vi "Fit VI window to Pane Center.vi"(4 "Error In":errorcluster, 6 "Pane Ref":refnum<vi>, 7 "VI Ref (calling VI)":refnum<vi>) -> (0 "Error Out":errorcluster, 3 "dup VI Ref":refnum<vi>)   [LabVIEW 2017]
doc: "This VI is designed to center a callee VI's window in a caller VI's window.\n\nAuthored by Brandon Steele\nsupport@mooregoodideas.com\nwww.mooregoodideas.com\n\nCopyright (c) 2010, Moore Good Ideas, Inc.\n\nAll rights reserved.\n\nRedistribution and use in source and binary forms, with or without modification, are permitted provided that the following conditions are met:\n\n * Redistributions of source code must retain the above copyright notice, this list of conditions and the following disclaimer.\n * Redistributions in binary form must reproduce the above copyright notice, this list of conditions and the following disclaimer in the documentation and/or other materials provided with the distribution.\n * Neither the name of Moore Good Ideas, Inc. nor the names of its contributors may be used to endorse or promote products derived from this software without specific prior written permission.\n\nTHIS SOFTWARE IS PROVIDED BY THE COPYRIGHT HOLDERS AND CONTRIBUTORS \"AS IS\" AND ANY EXPRESS OR IMPLIED WARRANTIES, INCLUDING, BUT NOT LIMITED TO, THE IMPLIED WARRANTIES OF MERCHANTABILITY AND FITNESS FOR A PARTICULAR PURPOSE ARE DISCLAIMED. IN NO EVENT SHALL THE COPYRIGHT OWNER OR CONTRIBUTORS BE LIABLE FOR ANY DIRECT, INDIRECT, INCIDENTAL, SPECIAL, EXEMPLARY, OR CONSEQUENTIAL DAMAGES (INCLUDING, BUT NOT LIMITED TO, PROCUREMENT OF SUBSTITUTE GOODS OR SERVICES; LOSS OF USE, DATA, OR PROFITS; OR BUSINESS INTERRUPTION) HOWEVER CAUSED AND ON ANY THEORY OF LIABILITY, WHETHER IN CONTRACT, STRICT LIABILITY, OR TORT (INCLUDING NEGLIGENCE OR OTHERWISE) ARISING IN ANY WAY OUT OF THE USE OF THIS SOFTWARE, EVEN IF ADVISED OF THE POSSIBILITY OF SUCH DAMAGE."
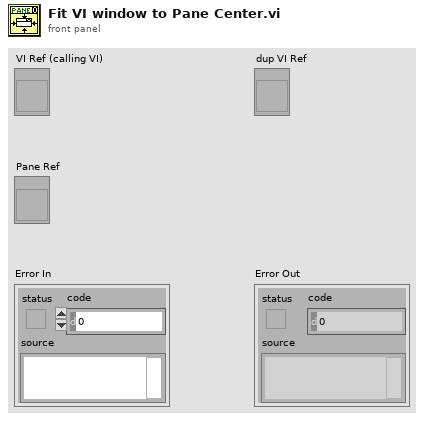
[diagram p1: front panel]
types:
  T1 = typedef "LVRectTypeDef.ctl" = cluster{"Left":i16, "Top":i16, "Right":i16, "Bottom":i16}
  T2 = cluster{"left":i16, "top":i16, "right":i16, "bottom":i16}
  T3 = typedef "LVAllMonitorsDisplayTypeDef.ctl" = cluster{"Bounds":cluster{"Left":i16, "Top":i16, "Right":i16, "Bottom":i16}, "Depth":i16}[]
  T4 = cluster{"Left":i16, "Top":i16, "Right":i16, "Bottom":i16}
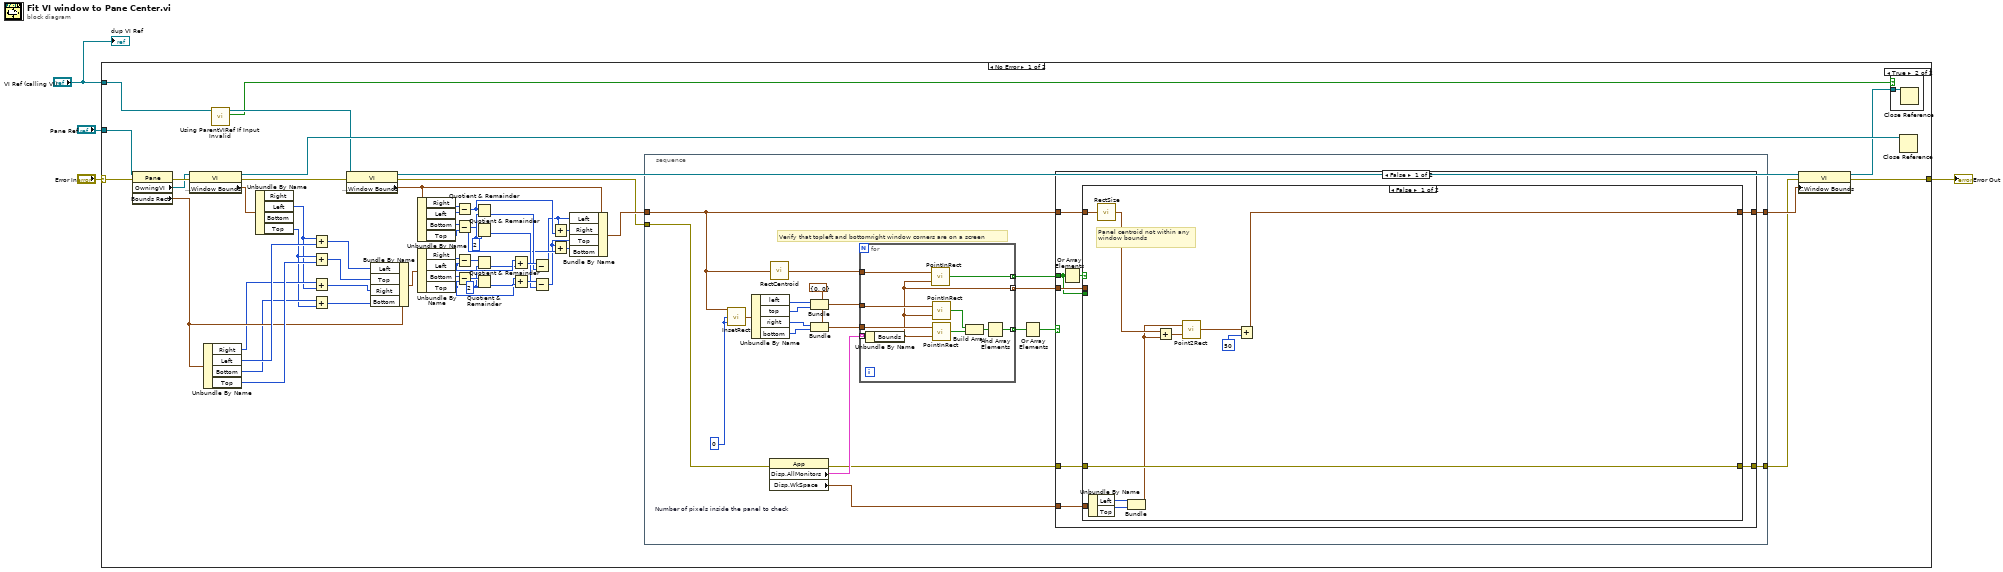
[diagram p0: block diagram]
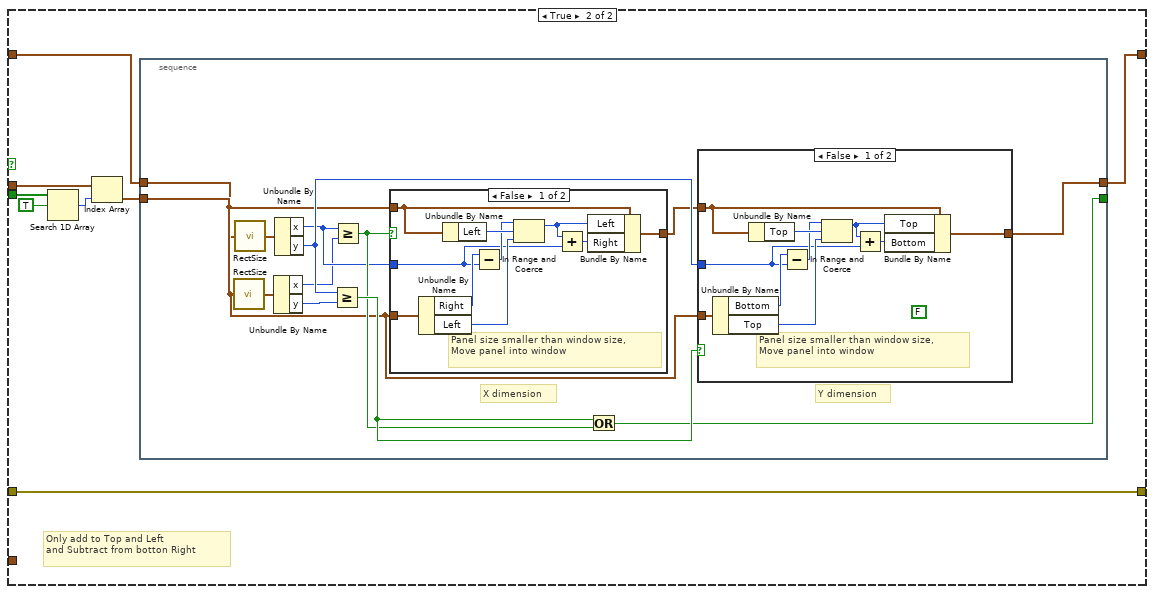
[diagram p2: hidden frame]
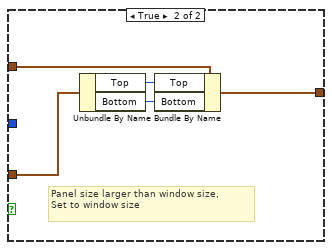
[diagram p3: hidden frame]
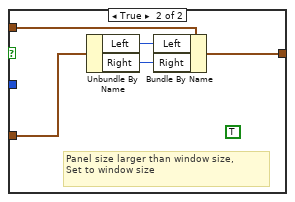
[diagram p4: hidden frame]
diagram:
  n1 = case shown="No Error" "Error In" {
    selector: "Error In" -> [w21 w163]
    tunnel: [w58 w163] -> w4
    tunnel: "Pane Ref" -> [w15 _]
    tunnel: "VI Ref (calling VI)" -> [w35 _]
    frame No Error {
      w52 = i16 2 ("y")
      w36 = i16 2 ("y")
      n2 = property class="Pane"(reference=w15, error in=w21) -> (error out=w20:errorcluster, "OwningVI"=w19:refnum<vi>, "Bounds Rect"=w12:T1)  [unwired: 1 out]
      n3 = property class="VI"(reference=w19, error in=w20) -> (reference out=w34:refnum<vi>, error out=w53:errorcluster, "Front Panel Window:Window Bounds"=w18:T1)
      n4 = Unbundle By Name(w12) -> ("Right"=w9:i16, "Left"=w14:i16, "Bottom"=w8:i16, "Top"=w13:i16)
      n5 = call "Using ParentVIRef If Input Invalid.vi"("VI Ref (calling VI)"=w35) -> ("Using Parent Ref(Need to Destroy)"=w24:bool, "VI Ref"=w32:refnum<vi>)  [unwired: 5 in]
      n6 = Unbundle By Name(w18) -> ("Left"=w6:i16, "Top"=w7:i16)  [unwired: 2 out]
      n7 = Add(x=w6, y=w14) -> (x+y=w17:i16)
      n8 = Add(x=w7, y=w13) -> (x+y=w16:i16)
      n9 = Add(x=w9, y=w6) -> (x+y=w11:i16)
      n10 = Add(x=w8, y=w7) -> (x+y=w10:i16)
      n11 = property class="VI"(reference=w32, error in=w53) -> (reference out=w39:refnum<vi>, error out=w23:errorcluster, "Front Panel Window:Window Bounds"=w27:T1)
      n12 = Bundle By Name(cluster=w12, "Left"=w17, "Top"=w16, "Right"=w11, "Bottom"=w10) -> (w5:T1)
      n13 = Unbundle By Name(w27) -> ("Right"=w48:i16, "Left"=w49:i16, "Bottom"=w50:i16, "Top"=w51:i16)
      n14 = Unbundle By Name(w5) -> ("Right"=w57:i16, "Left"=w47:i16, "Bottom"=w56:i16, "Top"=w44:i16)
      n15 = Subtract(x=w48, y=w49) -> (x-y=w38:i16)
      n16 = Subtract(x=w50, y=w51) -> (x-y=w37:i16)
      n17 = Subtract(x=w57, y=w47) -> (x-y=w55:i16)
      n18 = Subtract(x=w56, y=w44) -> (x-y=w54:i16)
      n19 = Quotient & Remainder(x=w38, y=w52) -> (floor(x/y)=w42:i16)  [unwired: 1 out]
      n20 = Quotient & Remainder(x=w37, y=w52) -> (floor(x/y)=w40:i16)  [unwired: 1 out]
      n21 = Quotient & Remainder(x=w55, y=w36) -> (floor(x/y)=w46:i16)  [unwired: 1 out]
      n22 = Quotient & Remainder(x=w54, y=w36) -> (floor(x/y)=w45:i16)  [unwired: 1 out]
      n23 = Add(x=w47, y=w46) -> (x+y=w43:i16)
      n24 = Add(x=w44, y=w45) -> (x+y=w41:i16)
      n25 = Subtract(x=w43, y=w42) -> (x-y=w30:i16)
      n26 = Subtract(x=w41, y=w40) -> (x-y=w29:i16)
      n27 = Add(x=w30, y=w38) -> (x+y=w28:i16)
      n28 = Add(x=w29, y=w37) -> (x+y=w31:i16)
      n29 = Bundle By Name(cluster=w27, "Left"=w30, "Right"=w28, "Top"=w29, "Bottom"=w31) -> (w26:T1)
      n30 = stacked-sequence {
        tunnel: [w69] -> w22
        tunnel: [w60] -> w25
        tunnel: w23 -> [w62]
        tunnel: w26 -> [w76]
        frame #0 {
          w71 = i16 0  # Number of pixels inside the panel to check
          w75 = cluster{"x":i16, "y":i16} {"x"=0, "y"=0} ("point")
          # "Verify that topleft and bottomright window corners are on a screen"
          n31 = call <vilib>:"InsetRect.vi"("dv"=w71, "dh"=w71, "rect"=w76) -> ("inset rect"=w65:T2)
          n32 = Unbundle By Name(w65) -> ("left"=w63:i16, "top"=w64:i16, "right"=w72:i16, "bottom"=w73:i16)
          n33 = property class="App"(error in=w62) -> (error out=w59:errorcluster, "Disp.AllMonitors"=w61:T3, "Disp.WkSpace"=w70:T1)  [unwired: 1 in, 1 out]
          n34 = call <vilib>:"RectCentroid.vi"("rect"=w76) -> ("point"=w77:cluster{"x":i16, "y":i16})
          n35 = Bundle(cluster=w75, "x"=w63, "y"=w64) -> (w66:cluster{"x":i16, "y":i16})
          n36 = Bundle(cluster=w75, "x"=w72, "y"=w73) -> (w74:cluster{"x":i16, "y":i16})
          n37 = for {
            tunnel: w61 -> [w161] mode=indexing
            tunnel: w66 -> [w160]
            tunnel: [w156] -> w67 mode=indexing
            tunnel: w74 -> [w155]
            tunnel: w77 -> [w154]
            tunnel: [w153] -> w78 mode=indexing
            tunnel: [w152] -> w79 mode=indexing
            n38 = Unbundle By Name(w161) -> ("Bounds"=w152:T4)
            n39 = call <vilib>:"PointInRect.vi"("rect"=w152, "point"=w154) -> ("pt in rect"=w153:bool)
            n40 = call <vilib>:"PointInRect.vi"("rect"=w152, "point"=w160) -> ("pt in rect"=w159:bool)
            n41 = call <vilib>:"PointInRect.vi"("rect"=w152, "point"=w155) -> ("pt in rect"=w158:bool)
            n42 = Build Array(w159, w158) -> (w157:bool[])
            n43 = And Array Elements(Boolean array=w157) -> (logical AND=w156:bool)
          }
          n44 = Or Array Elements(Boolean array=w67) -> (logical OR=w68:bool)
          n45 = case shown="False" w68 {
            tunnel: w59 -> [w82 w151]
            tunnel: [w81 w151] -> w69
            tunnel: w76 -> [w86 w150]
            tunnel: [w85 w150] -> w60
            tunnel: w70 -> [w87 _]
            tunnel: w78 -> [w80 _]
            tunnel: w79 -> [w83 _]
            frame False {
              n46 = Or Array Elements(Boolean array=w80) -> (logical OR=w84:bool)
              n47 = case shown="False" w84 {
                tunnel: w87 -> [w98 _]
                tunnel: w86 -> [w94 w101]
                tunnel: [w92 w99] -> w85
                tunnel: w83 -> [_ w103]
                tunnel: w82 -> [w91 w106]
                tunnel: [w91 w106] -> w81
                tunnel: w80 -> [_ w105]
                frame False {
                  # "Panel centroid not within any\nwindow bounds"
                  n48 = Unbundle By Name(w98) -> ("Left"=w97:i16, "Top"=w96:i16)
                  n49 = call <vilib>:"RectSize.vi"("rect"=w94) -> ("point"=w90:cluster{"x":i16, "y":i16})
                  n50 = Bundle("Left"=w97, "Top"=w96) -> (w88:cluster{"Left":i16, "Top":i16})  [unwired: 1 in]
                  n51 = Add(x=w90, y=w88) -> (x+y=w89:cluster{i16, i16})
                  n52 = call <vilib>:"Point2Rect.vi"("point b"=w89, "point a"=w88) -> ("rect"=w93:T2)
                  n53 = Add(x=w93, y=i16 50) -> (x+y=w92:T2)
                }
                frame True {
                  # "Only add to Top and Left\nand Subtract from botton Right"
                  n54 = Search 1D Array(1D array=w105, element=TRUE) -> (index of element=w102:i32)  [unwired: 1 in]
                  n55 = Index Array(array=w103, index=w102) -> (element=w100:T4)
                  n56 = stacked-sequence {
                    tunnel: [w107] -> _
                    tunnel: [w117] -> w99
                    tunnel: w100 -> [w116]
                    tunnel: w101 -> [w108]
                    frame #0 {
                      # "X dimension"
                      # "Y dimension"
                      n57 = call <vilib>:"RectSize.vi"("rect"=w116) -> ("point"=w110:cluster{"x":i16, "y":i16})
                      n58 = call <vilib>:"RectSize.vi"("rect"=w108) -> ("point"=w109:cluster{"x":i16, "y":i16})
                      n59 = Unbundle By Name(w110) -> ("x"=w111:i16, "y"=w114:i16)
                      n60 = Unbundle By Name(w109) -> ("x"=w112:i16, "y"=w115:i16)
                      n61 = Greater Or Equal?(x=w115, y=w114) -> (x >= y?=w119:bool)
                      n62 = Greater Or Equal?(x=w112, y=w111) -> (x >= y?=w118:bool)
                      n63 = case shown="False" w118 {
                        tunnel: w116 -> [w144 w145]
                        tunnel: w108 -> [w136 w146]
                        tunnel: w112 -> [w137 _]
                        tunnel: [w135 w147] -> w113
                        frame False {
                          # "Panel size smaller than window size,\nMove panel into window"
                          n64 = Unbundle By Name(w144) -> ("Right"=w140:i16, "Left"=w142:i16)
                          n65 = Unbundle By Name(w136) -> ("Left"=w143:i16)
                          n66 = Subtract(x=w140, y=w137) -> (x-y=w141:i16)
                          n67 = In Range and Coerce(upper limit=w141, x=w143, lower limit=w142) -> (coerced(x)=w139:i16)  [unwired: 1 out]
                          n68 = Add(x=w139, y=w137) -> (x+y=w138:i16)
                          n69 = Bundle By Name(cluster=w136, "Left"=w139, "Right"=w138) -> (w135:T1)
                        }
                        frame True {
                          (unwired) TRUE
                          # "Panel size larger than window size,\nSet to window size"
                          n70 = Unbundle By Name(w145) -> ("Left"=w149:i16, "Right"=w148:i16)
                          n71 = Bundle By Name(cluster=w146, "Left"=w149, "Right"=w148) -> (w147:T1)
                        }
                      }
                      n72 = Or(x=w119, y=w118) -> (x .or. y?=w107:bool)
                      n73 = case shown="False" w119 {
                        tunnel: w116 -> [w129 w134]
                        tunnel: w113 -> [w121 w130]
                        tunnel: w115 -> [w122 _]
                        tunnel: [w120 w131] -> w117
                        frame False {
                          (unwired) FALSE
                          # "Panel size smaller than window size,\nMove panel into window"
                          n74 = Unbundle By Name(w129) -> ("Bottom"=w125:i16, "Top"=w127:i16)
                          n75 = Unbundle By Name(w121) -> ("Top"=w128:i16)
                          n76 = Subtract(x=w125, y=w122) -> (x-y=w126:i16)
                          n77 = In Range and Coerce(upper limit=w126, x=w128, lower limit=w127) -> (coerced(x)=w124:i16)  [unwired: 1 out]
                          n78 = Add(x=w124, y=w122) -> (x+y=w123:i16)
                          n79 = Bundle By Name(cluster=w121, "Top"=w124, "Bottom"=w123) -> (w120:T1)
                        }
                        frame True {
                          # "Panel size larger than window size,\nSet to window size"
                          n80 = Unbundle By Name(w134) -> ("Top"=w133:i16, "Bottom"=w132:i16)
                          n81 = Bundle By Name(cluster=w130, "Top"=w133, "Bottom"=w132) -> (w131:T1)
                        }
                      }
                    }
                  }
                }
              }
            }
            frame True {
            }
          }
        }
      }
      n82 = property class="VI"(reference=w39, error in=w22, "Front Panel Window:Window Bounds"=w25) -> (reference out=w33:refnum<vi>, error out=w58:errorcluster)
      n83 = case shown="True" w24 {
        tunnel: w33 -> [_ w162]
        frame False {
        }
        frame True {
          n84 = Close Reference(reference=w162) -> ()  [unwired: 1 in, 1 out]
        }
      }
      n85 = Close Reference(reference=w34) -> ()  [unwired: 1 in, 1 out]
    }
    frame Error {
    }
  }
  "Error Out" <- w4
  "dup VI Ref" <- "VI Ref (calling VI)"
